vi "SaveOdorInf.vi"(9 "Path":path, 10 "Concentrations":string[](array[string]), 11 "Odors":string[](array[string])) -> ()   [LabVIEW 2016]
uses:
  <vilib>/Utility/file.llb/Write Delimited Spreadsheet (string).vi
panel:
  out "file created?":bool
  out "error in (no error)":errorcluster
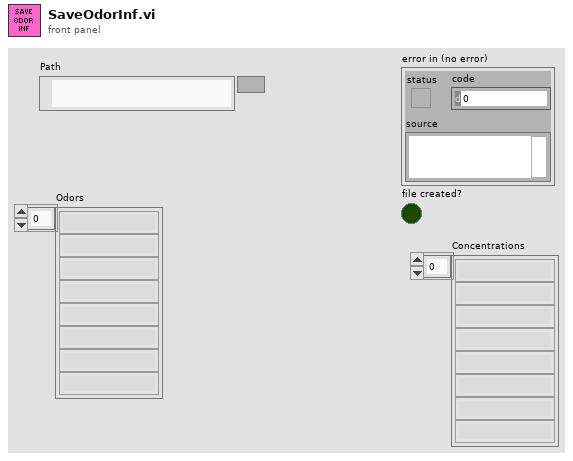
[diagram p1: front panel]
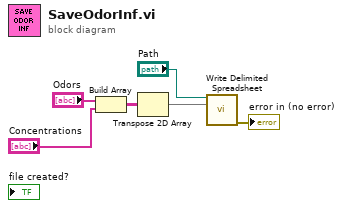
[diagram p0: block diagram]
diagram:
  n1 = Build Array("Odors", "Concentrations") -> (w4:string[][])
  n2 = Transpose 2D Array(2D array=w4) -> (transposed array=w1:string[][])
  n3 = call-poly <vilib>:"Write Delimited Spreadsheet.vi"("file path (dialog if empty)"="Path", "2D data"=w1) -> ("error out"=→"error in (no error)":errorcluster)  [unwired: 12 in, 1 out]
